vi "Color Picker_Color to Hue Sat Lum.vi"(8 "Error In":errorcluster, 11 "Color Box":u32(colorbox)) -> (0 "Error Out":errorcluster, 3 "Color Value Out":T1)   [LabVIEW 2009]
doc: "Seperates color into the Hue, Saturation and Luminance components"
uses:
  Color Picker Controls/Color Picker_Cluster Color Component Data Set.ctl
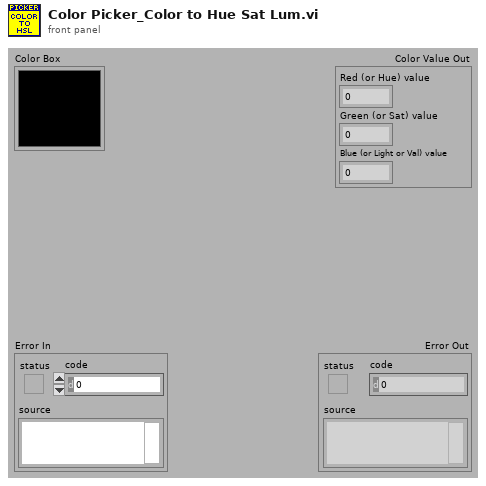
[diagram p1: front panel]
types:
  T1 = typedef "Color Picker_Cluster Color Component Data Set.ctl" = cluster{"Blue (or Light or Val) value":u8, "Green (or Sat) value":u8, "Red (or Hue) value":u8}
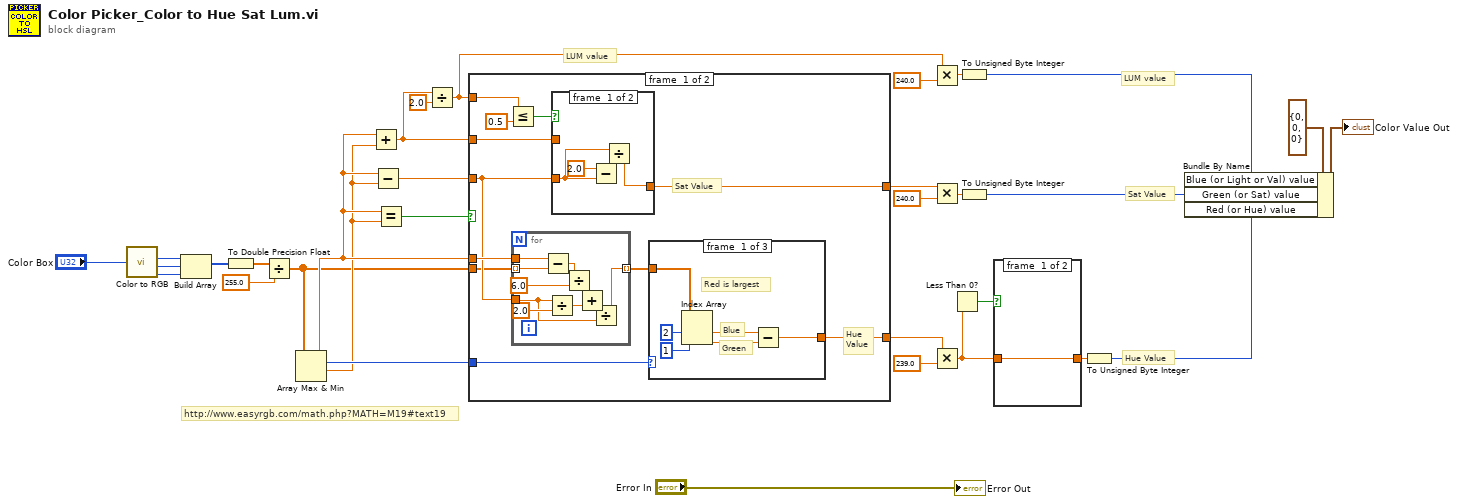
[diagram p0: block diagram]
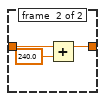
[diagram p2: hidden frame]
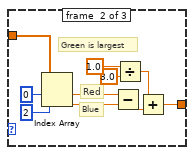
[diagram p3: hidden frame]
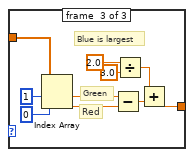
[diagram p4: hidden frame]
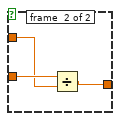
[diagram p5: hidden frame]
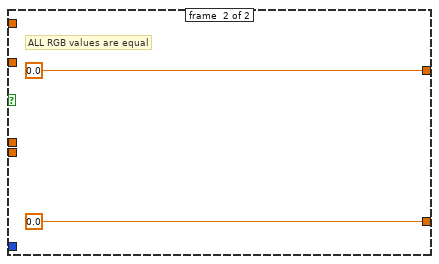
[diagram p6: hidden frame]
diagram:
  # "Sat Value"
  # "LUM value"
  # "Hue Value"
  # "http://www.easyrgb.com/math.php?MATH=M19#text19"
  # "LUM value"
  n1 = call <vilib>:"Color to RGB.vi"("Color"="Color Box") -> ("R"=w31:u8, "G"=w30:u8, "B"=w29:u8)  [unwired: 1 out]
  n2 = Build Array(w31, w30, w29) -> (w28:u8[])
  n3 = To Double Precision Float(number=w28) -> (double precision float=w27:dbl[])
  n4 = Divide(x=w27, y=255.0) -> (x/y=w18:dbl[])
  n5 = Array Max & Min(array=w18) -> (max value=w22:dbl, max index (indices)=w23:i32, min value=w21:dbl)  [unwired: 1 out]
  n6 = Add(x=w22, y=w21) -> (x+y=w20:dbl)
  n7 = Subtract(x=w22, y=w21) -> (x-y=w19:dbl)
  n8 = Equal?(x=w22, y=w21) -> (x = y?=w24:bool)
  n9 = Divide(x=w20, y=2.0) -> (x/y=w10:dbl)
  n10 = case shown="False" w24 {
    tunnel: w22 -> [w36 _]
    tunnel: w23 -> [w38 _]
    tunnel: w10 -> [w42 _]
    tunnel: w20 -> [w40 _]
    tunnel: w19 -> [w35 _]
    tunnel: [w39 0.0] -> w17
    tunnel: w18 -> [w34 _]
    tunnel: [w37 0.0] -> w14
    frame #0 {
      # "Hue\nValue"
      # "Sat Value"
      n11 = Less Or Equal?(x=w42, y=0.5) -> (x <= y?=w41:bool)
      n12 = for {
        tunnel: w34 -> [w52] mode=indexing
        tunnel: w36 -> [w53]
        tunnel: w35 -> [w45]
        tunnel: [w44] -> w33 mode=indexing
        n13 = Subtract(x=w53, y=w52) -> (x-y=w51:dbl)
        n14 = Divide(x=w45, y=2.0) -> (x/y=w47:dbl)
        n15 = Divide(x=w51, y=6.0) -> (x/y=w48:dbl)
        n16 = Add(x=w48, y=w47) -> (x+y=w46:dbl)
        n17 = Divide(x=w46, y=w45) -> (x/y=w44:dbl)
      }
      n18 = case shown="False" w41 {
        tunnel: w35 -> [w82 w86]
        tunnel: w40 -> [_ w85]
        tunnel: [w80 w84] -> w39
        frame #0 {
          n19 = Subtract(x=2.0, y=w82) -> (x-y=w81:dbl)
          n20 = Divide(x=w82, y=w81) -> (x/y=w80:dbl)
        }
        frame #1 {
          n21 = Divide(x=w86, y=w85) -> (x/y=w84:dbl)
        }
      }
      n22 = case shown="0, Default" w38 {
        tunnel: w33 -> [w59 w69 w79]
        tunnel: [w54 w64 w74] -> w37
        frame #0 {
          # "Blue"
          # "Green"
          # "Red is largest"
          n23 = Index Array(array=w59, index #1=2 ("index"), index #2=1 ("index")) -> (element #1=w56:dbl, element #2=w55:dbl)
          n24 = Subtract(x=w56, y=w55) -> (x-y=w54:dbl)
        }
        frame #1 {
          # "Red"
          # "Blue"
          # "Green is largest"
          n25 = Index Array(array=w69, index #1=0 ("index"), index #2=2 ("index")) -> (element #1=w66:dbl, element #2=w65:dbl)
          n26 = Subtract(x=w66, y=w65) -> (x-y=w60:dbl)
          n27 = Divide(x=1.0, y=3.0) -> (x/y=w61:dbl)
          n28 = Add(x=w61, y=w60) -> (x+y=w64:dbl)
        }
        frame #2 {
          # "Green"
          # "Red"
          # "Blue is largest"
          n29 = Index Array(array=w79, index #1=1 ("index"), index #2=0 ("index")) -> (element #1=w76:dbl, element #2=w75:dbl)
          n30 = Subtract(x=w76, y=w75) -> (x-y=w70:dbl)
          n31 = Divide(x=2.0, y=3.0) -> (x/y=w71:dbl)
          n32 = Add(x=w71, y=w70) -> (x+y=w74:dbl)
        }
      }
    }
    frame #1 {
      # "ALL RGB values are equal"
    }
  }
  n33 = Multiply(x=w10, y=240.0) -> (x*y=w12:dbl)
  n34 = Multiply(x=w17, y=240.0) -> (x*y=w13:dbl)
  n35 = Multiply(x=w14, y=239.0) -> (x*y=w3:dbl)
  n36 = Less Than 0?(x=w3) -> (x < 0?=w9:bool)
  n37 = To Unsigned Byte Integer(number=w12) -> (unsigned 8bit integer=w5:u8)
  n38 = To Unsigned Byte Integer(number=w13) -> (unsigned 8bit integer=w6:u8)
  n39 = case shown="True" w9 {
    tunnel: w3 -> [w89 w92]
    tunnel: [w89 w90] -> w4
    frame #0 {
    }
    frame #1 {
      n40 = Add(x=w92, y=240.0) -> (x+y=w90:dbl)
    }
  }
  n41 = To Unsigned Byte Integer(number=w4) -> (unsigned 8bit integer=w2:u8)
  n42 = Bundle By Name(cluster=T1 {"Blue (or Light or Val) value"=0, "Green (or Sat) value"=0, "Red (or Hue) value"=0} ("Color Value"), "Blue (or Light or Val) value"=w5, "Green (or Sat) value"=w6, "Red (or Hue) value"=w2) -> (→"Color Value Out":T1)
  "Error Out" <- "Error In"
